vi "Aux DMA derived clock test.vi"() -> ()   [LabVIEW 2019]
uses:
  <vilib>/Platform/TimedLoop/XDataNode/timing_clust.ctl
  <vilib>/Platform/TimedLoop/XDataNode/nitl_modes.ctl
  <vilib>/Platform/TimedLoop/XDataNode/wakeup.ctl
  <vilib>/rvi/Emulation/niFpgaSctlEmulationGetInTimedLoop.vi
  <vilib>/rvi/Emulation/niFpgaEmulationReportErrorSimple.vi
  <vilib>/rvi/Emulation/niFpgaGetClockAttributes.vi
  <vilib>/rvi/Emulation/niFpgaCriticalErrorInLSC.vi
  <vilib>/rvi/eio/common/nirviEmuTemplateMethod_errors.vi
  <vilib>/rvi/interface/RandomDataEmulation/niFpgaRandomDataHandleErrors.vi
  <vilib>/platform/TimedLoop/XDataNode/XDataNode.xnode
  <vilib>/eio/EIONode/EIONode.xnode
  <vilib>/rvi/DataTransferAndStorage/Container/XNode/niFpgaContainer.xnode
  <vilib>/rvi/interface/RandomDataEmulation/nirviRandomDataFpgaReadWriteTemplate.vi
  <vilib>/Platform/TimedLoop/XDataNode/XDNodeRunTimeDep.lvlib
panel:
  in  "aux_portlist_0":u16[](array[numeric])=[0, 0, 0, 0, 0, 0]
  out "port FIFO state":enum8{"reading", "waiting"}(ring)
  in  "xt end aux":u32
  out "elapsed":u32
  out "xt counter":u32
  in  "xt total":u32
  out "xt success":bool
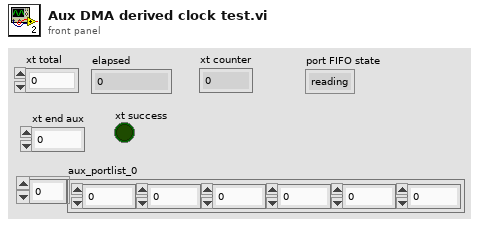
[diagram p1: front panel]
types:
  T1 = typedef "XDNodeRunTimeDep.lvlib/timing_clust.ctl" = cluster{"Expected End [f-1]":u64, "Actual End [f-1]":u64, "Finished Late? [f-1]":bool, "Expected End [i-1]":u64, "Actual End [i-1]":u64, "Finished Late? [i-1]":bool, "Expected Start [i]":u64, "Actual Start [i]":u64, "Expected Start [f]":u64, "Actual Start [f]":u64, "Source Name":string, "Structure Name":string, "Period":i64, "Deadline":i64, "Offset":i64, "Start":i64, "Priority":i32, "Timeout":i32, "Mode":T2, "Wakeup Reason":T3, "Error":errorcluster, "Source Type":string, "Secondary Source Type":string, "Global End Time":u64, "Global Start Time":u64, "Frame Duration":u64, "Iteration Duration":u64, "Assigned CPU":i32, "I/O Scan Engine Mode":u32}
  T2 = typedef "XDNodeRunTimeDep.lvlib/nitl_modes.ctl" = enum32{"No Change", "Process missed periods, maintain original phase", "Discard missed periods, maintain original phase", "Process missed periods, ignore original phase", "Discard missed periods, ignore original phase"}
  T3 = typedef "XDNodeRunTimeDep.lvlib/wakeup.ctl" = enum32{"Normal", "Aborted", "Asynchronous wakeup", "Timing source error", "Timed loop error", "Timeout"}
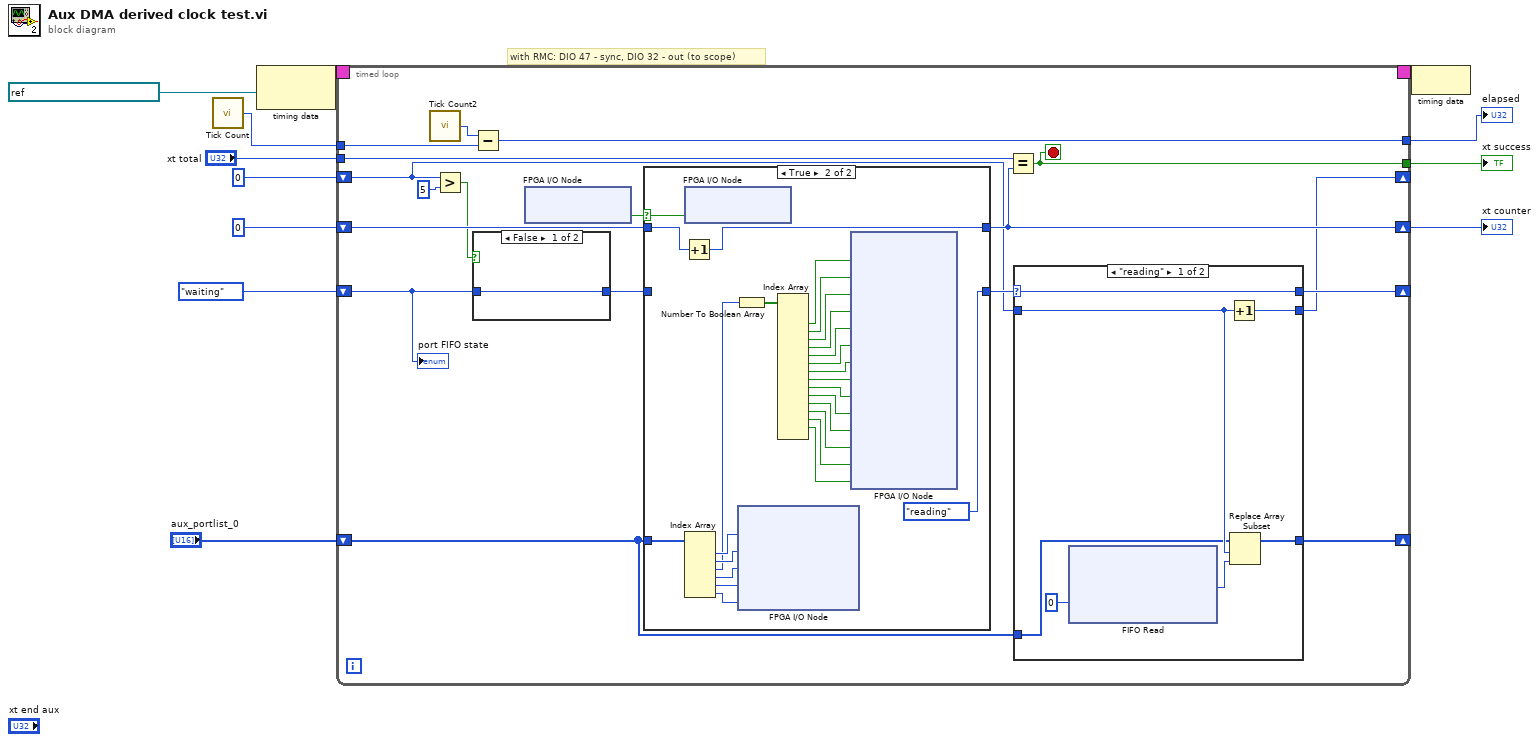
[diagram p0: block diagram]
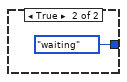
[diagram p2: hidden frame]
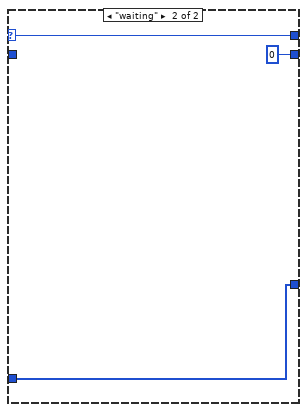
[diagram p3: hidden frame]
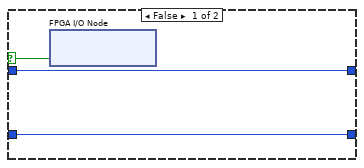
[diagram p4: hidden frame]
diagram:
  # "with RMC: DIO 47 - sync, DIO 32 - out (to scope)"
  n1 = call "Tick Count"() -> ("Tick Count(uSec)"=w10:u32)
  n2 = node-c288(refnum<k21> "40 MHz Onboard Clock" ("Source Name")) -> (w12:T1)
  n3 = timed-loop {
    tunnel: w10 -> [w30]
    tunnel: [w28] -> w9
    shift-right: [w24] -> w8
    shift-left: u32 0 -> [w25]
    timing: w12 -> [_]
    timing-out: [_] -> w11
    tunnel: "xt total" -> [w23]
    tunnel: [w26] -> w4
    shift-right: [w22] -> _
    shift-left: enum8{"reading", "waiting"}."waiting" -> [w17]
    shift-right: [w14] -> _
    shift-left: u8 0 -> [w15]
    shift-right: [w13] -> _
    shift-left: "aux_portlist_0" -> [w16]
    stop <- w26 stop-if-true
    n4 = call "Tick Count2"() -> ("Tick Count(uSec)"=w29:u32)
    n5 = Greater?(x=w15, y=u8 5) -> (0:w20:bool)
    n6 = Subtract(x=w29, y=w30) -> (x-y=w28:u32)
    n7 = case shown="False" w20 {
      tunnel: [w31 enum8{"reading", "waiting"}."waiting"] -> w18
      tunnel: w17 -> [w31 _]
      frame False {
      }
      frame True {
      }
    }
    n8 = xnode "FPGA I/O Node"() -> ("RMC/DIO47"=w27:bool)  [unwired: 1 in, 1 out]
    n9 = case shown="True" w27 {
      selector: w27 -> [w44 w69]
      tunnel: w25 -> [w45 w71]
      tunnel: [w45 w70] -> w24
      tunnel: [w43 enum8{"reading", "waiting"}."reading"] -> w21
      tunnel: w18 -> [w43 _]
      tunnel: w16 -> [_ w52]
      frame False {
        n10 = xnode "FPGA I/O Node"("RMC/DIO32"=w44) -> ()  [unwired: 1 in, 1 out]
      }
      frame True {
        n11 = Increment(x=w71) -> (x+1=w70:u32)
        n12 = xnode "FPGA I/O Node"("RMC/DIO32"=w69) -> ()  [unwired: 1 in, 1 out]
        n13 = Index Array(array=w52) -> (element #1=w51:u16, element #2=w50:u16, element #3=w49:u16, element #4=w48:u16, element #5=w47:u16, element #6=w46:u16)  [unwired: 6 in]
        n14 = Number To Boolean Array(number=w49) -> (Boolean array=w67:bool[])
        n15 = xnode "FPGA I/O Node"("RMC/DIO15:0"=w51, "RMC/DIO31:16"=w50, "RMC/DIO63:48"=w48, "RMC/DIO79:64"=w47, "RMC/DIO95:80"=w46) -> ()  [unwired: 5 in, 5 out]
        n16 = Index Array(array=w67) -> (element #2=w66:bool, element #3=w65:bool, element #4=w64:bool, element #5=w63:bool, element #6=w62:bool, element #7=w61:bool, element #8=w60:bool, element #9=w59:bool, element #10=w58:bool, element #11=w57:bool, element #12=w56:bool, element #13=w55:bool, element #14=w54:bool, element #15=w53:bool)  [unwired: 16 in, 2 out]
        n17 = xnode "FPGA I/O Node"("RMC/DIO33"=w66, "RMC/DIO34"=w65, "RMC/DIO35"=w64, "RMC/DIO36"=w63, "RMC/DIO37"=w62, "RMC/DIO38"=w61, "RMC/DIO39"=w60, "RMC/DIO40"=w59, "RMC/DIO41"=w58, "RMC/DIO42"=w57, "RMC/DIO43"=w56, "RMC/DIO44"=w55, "RMC/DIO45"=w54, "RMC/DIO46"=w53) -> ()  [unwired: 14 in, 14 out]
      }
    }
    n18 = Equal?(x=w23, y=w24) -> (x = y?=w26:bool)
    n19 = case shown="\"reading\"" w21 {
      selector: w21 -> [w38 w42]
      tunnel: [w38 w42] -> w22
      tunnel: w16 -> [w34 w41]
      tunnel: w15 -> [w36 _]
      tunnel: [w35 u8 0] -> w14
      tunnel: [w33 w41] -> w13
      frame "reading" {
        n20 = xnode ("FIFO Read")("Timeout"=0) -> ("Element"=w37:u16)  [unwired: 1 in, 2 out]
        n21 = Increment(x=w36) -> (x+1=w35:u8)
        n22 = Replace Array Subset(array=w34, new element=w37, index=w36) -> (w33:u16[])
      }
      frame "waiting" {
      }
    }
    "port FIFO state" <- w17
  }
  "elapsed" <- w9
  "xt counter" <- w8
  "xt success" <- w4
  n23 = node-c288(w11) -> ()
